vi "Logging Stringify Entry Value.vi"(1 "Entry":T1) -> (0 "String":string)   [LabVIEW 2012, in "femtoRoboLib.lvlib"]
uses:
  Log Entry.ctl
  Log Value Type.ctl
  Log Value Cluster.ctl
  femtoRoboLib.lvlib
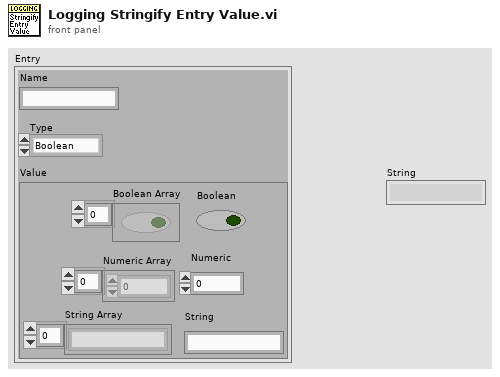
[diagram p1: front panel]
types:
  T1 = typedef "femtoRoboLib.lvlib/Log Entry.ctl" = cluster{"Name":string, "Type":T2, "Value":T3}
  T2 = typedef "femtoRoboLib.lvlib/Log Value Type.ctl" = enum16{"Boolean", "Numeric", "String", "Boolean Array", "Numeric Array", "String Array"}
  T3 = typedef "femtoRoboLib.lvlib/Log Value Cluster.ctl" = cluster{"Boolean Array":bool[], "Boolean":bool, "Numeric Array":dbl[], "Numeric":dbl, "String Array":string[], "String":string}
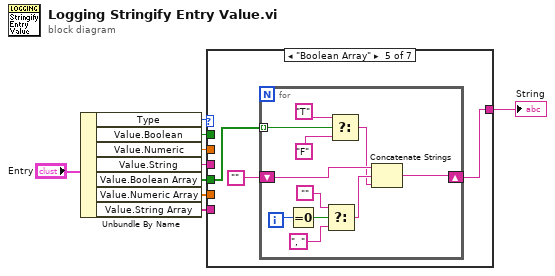
[diagram p0: block diagram]
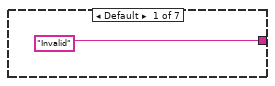
[diagram p2: hidden frame]
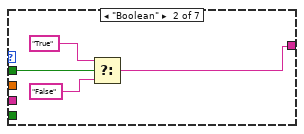
[diagram p3: hidden frame]
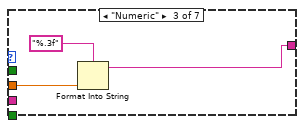
[diagram p4: hidden frame]
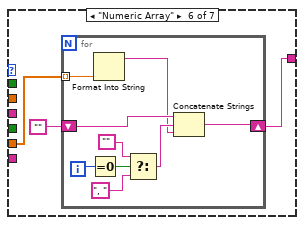
[diagram p6: hidden frame]
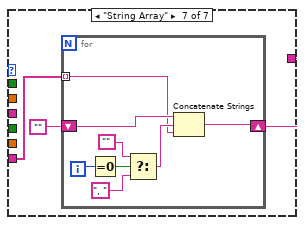
[diagram p7: hidden frame]
diagram:
  n1 = Unbundle By Name("Entry") -> ("Type"=w7:T2, "Value.Boolean"=w6:bool, "Value.Numeric"=w5:dbl, "Value.String"=w4:string, "Value.Boolean Array"=w3:bool[], "Value.Numeric Array"=w2:dbl[], "Value.String Array"=w1:string[])
  n2 = case shown="\"Boolean Array\"" w7 {
    tunnel: ["Invalid" w12 w17 w18 w20 w34 w46] -> w9
    tunnel: w6 -> [_ w11 _ _ _ _ _]
    tunnel: w5 -> [_ _ w15 _ _ _ _]
    tunnel: w4 -> [_ _ _ w18 _ _ _]
    tunnel: w3 -> [_ _ _ _ w19 _ _]
    tunnel: w2 -> [_ _ _ _ _ w33 _]
    tunnel: w1 -> [_ _ _ _ _ _ w45]
    frame Default {
    }
    frame "Boolean" {
      n3 = Select(t="True", s=w11, f="False") -> (s? t:f=w12:string)
    }
    frame "Numeric" {
      n4 = Format Into String(format string="%.3f", w15) -> (resulting string=w17:string)  [unwired: 2 in, 1 out]
    }
    frame "String" {
    }
    frame "Boolean Array" {
      n5 = for {
        tunnel: w19 -> [w30] mode=indexing
        shift-right: [w23] -> w20
        shift-left: "" -> [w29]
        i -> [w28]
        n6 = Equal To 0?(x=w28) -> (x = 0?=w27:bool)
        n7 = Select(t="", s=w27, f=", ") -> (s? t:f=w24:string)
        n8 = Select(t="T", s=w30, f="F") -> (s? t:f=w22:string)
        n9 = Concatenate Strings(w29, w24, w22) -> (w23:string)
      }
    }
    frame "Numeric Array" {
      n10 = for {
        tunnel: w33 -> [w37] mode=indexing
        shift-right: [w38] -> w34
        shift-left: "" -> [w44]
        i -> [w43]
        n11 = Equal To 0?(x=w43) -> (x = 0?=w42:bool)
        n12 = Format Into String(w37) -> (resulting string=w36:string)  [unwired: 3 in, 1 out]
        n13 = Select(t="", s=w42, f=", ") -> (s? t:f=w39:string)
        n14 = Concatenate Strings(w44, w39, w36) -> (w38:string)
      }
    }
    frame "String Array" {
      n15 = for {
        tunnel: w45 -> [w48] mode=indexing
        shift-right: [w49] -> w46
        shift-left: "" -> [w55]
        i -> [w54]
        n16 = Equal To 0?(x=w54) -> (x = 0?=w53:bool)
        n17 = Select(t="", s=w53, f=", ") -> (s? t:f=w50:string)
        n18 = Concatenate Strings(w55, w50, w48) -> (w49:string)
      }
    }
  }
  "String" <- w9
